vi "Periodic Tasks.vi"(8 "error in":errorcluster) -> ()   [LabVIEW 2015]
doc: "This VI runs in parallel to other tasks. It can contain as many user-defined periodic loops as you need. These can carry out PID or other sorts of timed response."
uses:
  <vilib>/Rock Robotics/WPI/RobotDrive/WPI_RobotDriveMotorSelectorEnum.ctl
  <vilib>/Rock Robotics/WPI/CAN/TalonSRX/WPI_CANTalonSRX_APIFeedbackSelect.ctl
  <vilib>/Rock Robotics/WPI/Utilities/WPI_GetSetVariantRefNum.vi
  Sensors.vi
panel:
  out "x/y":dbl(graph)=0.002857142857142857
  in  "VISA resource name":refnum<visa-resource-name>="FTDI"
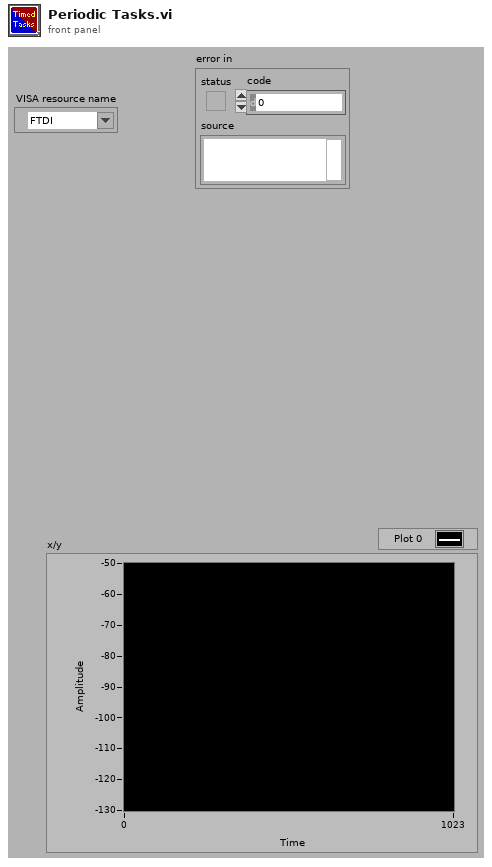
[diagram p1: front panel]
types:
  T1 = typedef "WPI_CANTalonSRX_APIFeedbackSelect.ctl" = enum16{"Digital Quadrature Encoder", "Analog Potentiometer", "Analog Encoder", "Count on Quad-A (Rising-Edge)", "Count on Quad-A (Falling-Edge)", "CTR Magnetic Enc (Absolute)", "CTR Magnetic Enc (Relative)", "Pulse Width"}
  T2 = typedef "WPI_RobotDriveMotorSelectorEnum.ctl" = enum16{"Rear Left Motor", "Rear Right Motor", "Front Left Motor", "Front Right Motor"}
  T3 = typedef "WPI_RobotDriveDevRef.ctl" = cluster{"DevStatus":errorcluster, "Motors[]":T4[], "Square Inputs":bool, "Max Output":dbl}
  T4 = typedef "WPI_MotorControlDeviceRef.ctl" = cluster{"DeviceStatus":errorcluster, "Type":T5, "PWM":cluster{"PWM Channel":T6, "DeadBand":T7}, "CAN":cluster{"Device Number":u8, "Control Mode":T8, "Semaphore":T9, "Max Vout":dbl, "TalonSRX Control Mode":T10}, "Invert":bool}
  T5 = typedef "WPI_MotorControlType.ctl" = enum16{"PWM", "CAN", "CANTalonSRX"}
  T6 = typedef "FPGA_DIOPWMChannel.ctl" = enum8{"PWM 0", "PWM 1", "PWM 2", "PWM 3", "PWM 4", "PWM 5", "PWM 6", "PWM 7", "PWM 8", "PWM 9", "PWM MXP 0", "PWM MXP 1", "PWM MXP 2", "PWM MXP 3", "PWM MXP 4", "PWM MXP 5", "PWM MXP 6", "PWM MXP 7", "PWM MXP 8", "PWM MXP 9", "Invalid"}
  T7 = typedef "WPI_PWMDeadband.ctl" = cluster{"Name":string, "maxPositivePwm":i32, "minPositivePwm":i32, "centerPwm":i32, "maxNegativePwm":i32, "minNegativePwm":i32, "angularRange":u16}
  T8 = typedef "WPI_CANJaguar_ControlMode.ctl" = enum8{"Percent VBus", "Current", "Speed", "Position", "Voltage"}
  T9 = typedef "Semaphore RefNum" = refnum<k1>
  T10 = typedef "WPI_CANTalonSRX_APIControlMode.ctl" = enum8{"Percent VBus", "Speed", "Position", "Slave", "Unchanged / Invalid", "Voltage Compensation", "Current", "Motion Profile"}
  T11 = typedef "WPI_JoystickDevRef.ctl" = cluster{"Device":T12}
  T12 = typedef "WPI_JoystickDeviceEnum.ctl" = enum16{"USB 0", "USB 1", "USB 2", "USB 3", "USB 4", "USB 5"}
  T13 = cluster{"JoystickDevRef":T11, "RobotDriveDevRef":T3}
  T14 = typedef "WPI_AccelerometerDevRef.ctl" = cluster{"DevStatus":errorcluster, "Scaling":T15, "Analog Channels":T16, "I2C Bus":T18, "SPI Bus":T19, "Accel Range":T20, "ADXL Axes":T21, "Handle":i32, "Device Address":u8, "Accel Type":enum16{"Analog", "ADXL345 I2C", "ADXL345 SPI", "Internal", "ADXL362 SPI"}}
  T15 = typedef "WPI_AccelerometerScaling.ctl" = cluster{"Gain (VoltsPerG)":dbl, "Center Voltage":dbl}
  T16 = typedef "WPI_AccelerometerAnalogChannels.ctl" = cluster{"X-Axis":T17, "Y-Axis":T17, "Z-Axis":T17}
  T17 = typedef "FPGA_AIChannel.ctl" = enum8{"AI 0", "AI 1", "AI 2", "AI 3", "AI MXP 0", "AI MXP 1", "AI MXP 2", "AI MXP 3", "Invalid"}
  T18 = typedef "i2c_bus.ctl" = enum16{"I2C On-Board", "I2C MXP", "Invalid"}
  T19 = typedef "spi_bus.ctl" = enum16{"SPI On-Board, CS0", "SPI On-Board, CS1", "SPI On-Board, CS2", "SPI On-Board, CS3", "SPI MXP", "Invalid"}
  T20 = typedef "ADXL345 Range.ctl" = u8
  T21 = typedef "WPI_AccelerometerADXL345 Axes.ctl" = cluster{"X-Axis":bool, "Y-Axis":bool, "Z-Axis":bool}
  T22 = typedef "WPI_CANTalonSRX_GlobalStatus.ctl" = cluster{"Applied Throttle":dbl, "Module Enabled":bool, "CAN Error":errorcluster, "Closed Loop Error":dbl, "Forward Limit Switch Closed":bool, "Reverse Limit Switch Closed":bool, "Sensor Position":dbl, "Sensor Velocity":dbl, "Current":dbl, "Sticky Fault - Over Temp":bool, "Sticky Fault - Under Voltage":bool, "Sticky Fault - Forward Limit":bool, "Sticky Fault - Reverse Limit":bool, "Sticky Fault - Forward Soft Limit":bool, "Sticky Fault - Reverse Soft Limit":bool, "Brake is Enabled":bool, "Encoder Position":dbl, "Encoder Velocity":dbl, "Encoder Index Count":dbl, "Encoder A Pin State":bool, "Encoder B Pin State":bool, "Encoder Index Pin State":bool, "Analog In":dbl, "Analog In Velocity":dbl, "Temperature (C)":dbl, "Battery Voltage":dbl, "Control 5 Is Supported":bool, "Current Profile Slot Select":dbl, "Pos Div 8":bool, "Vel Div 4":bool, "Pulse Width Position":i32, "Pulse Width Velocity":i32, "Pulse Width Rise To Rise (us)":i32, "Pulse Width Rise To Fall (us)":i32, "Mot Prof Active Is Under Run":bool, "Mot Prof Active Has Under Run":bool, "Mot Prof Active Is Last":bool, "Mot Prof Active Velocity Only":bool, "Mot Prof Active Is Valid":bool, "Mot Prof Buffer Is Full":bool, "Mot Prof Active Profile Slot Select":i32, "Mot Prof NextID":i32, "Mot Prof Count":i32, "Mot Prof Active Velocity":dbl, "Mot Prof Active Position":dbl, "Mot Prof Output Enable":i32}
  T23 = cluster{"X-Axis":dbl, "Y-Axis":dbl, "Z-Axis":dbl}
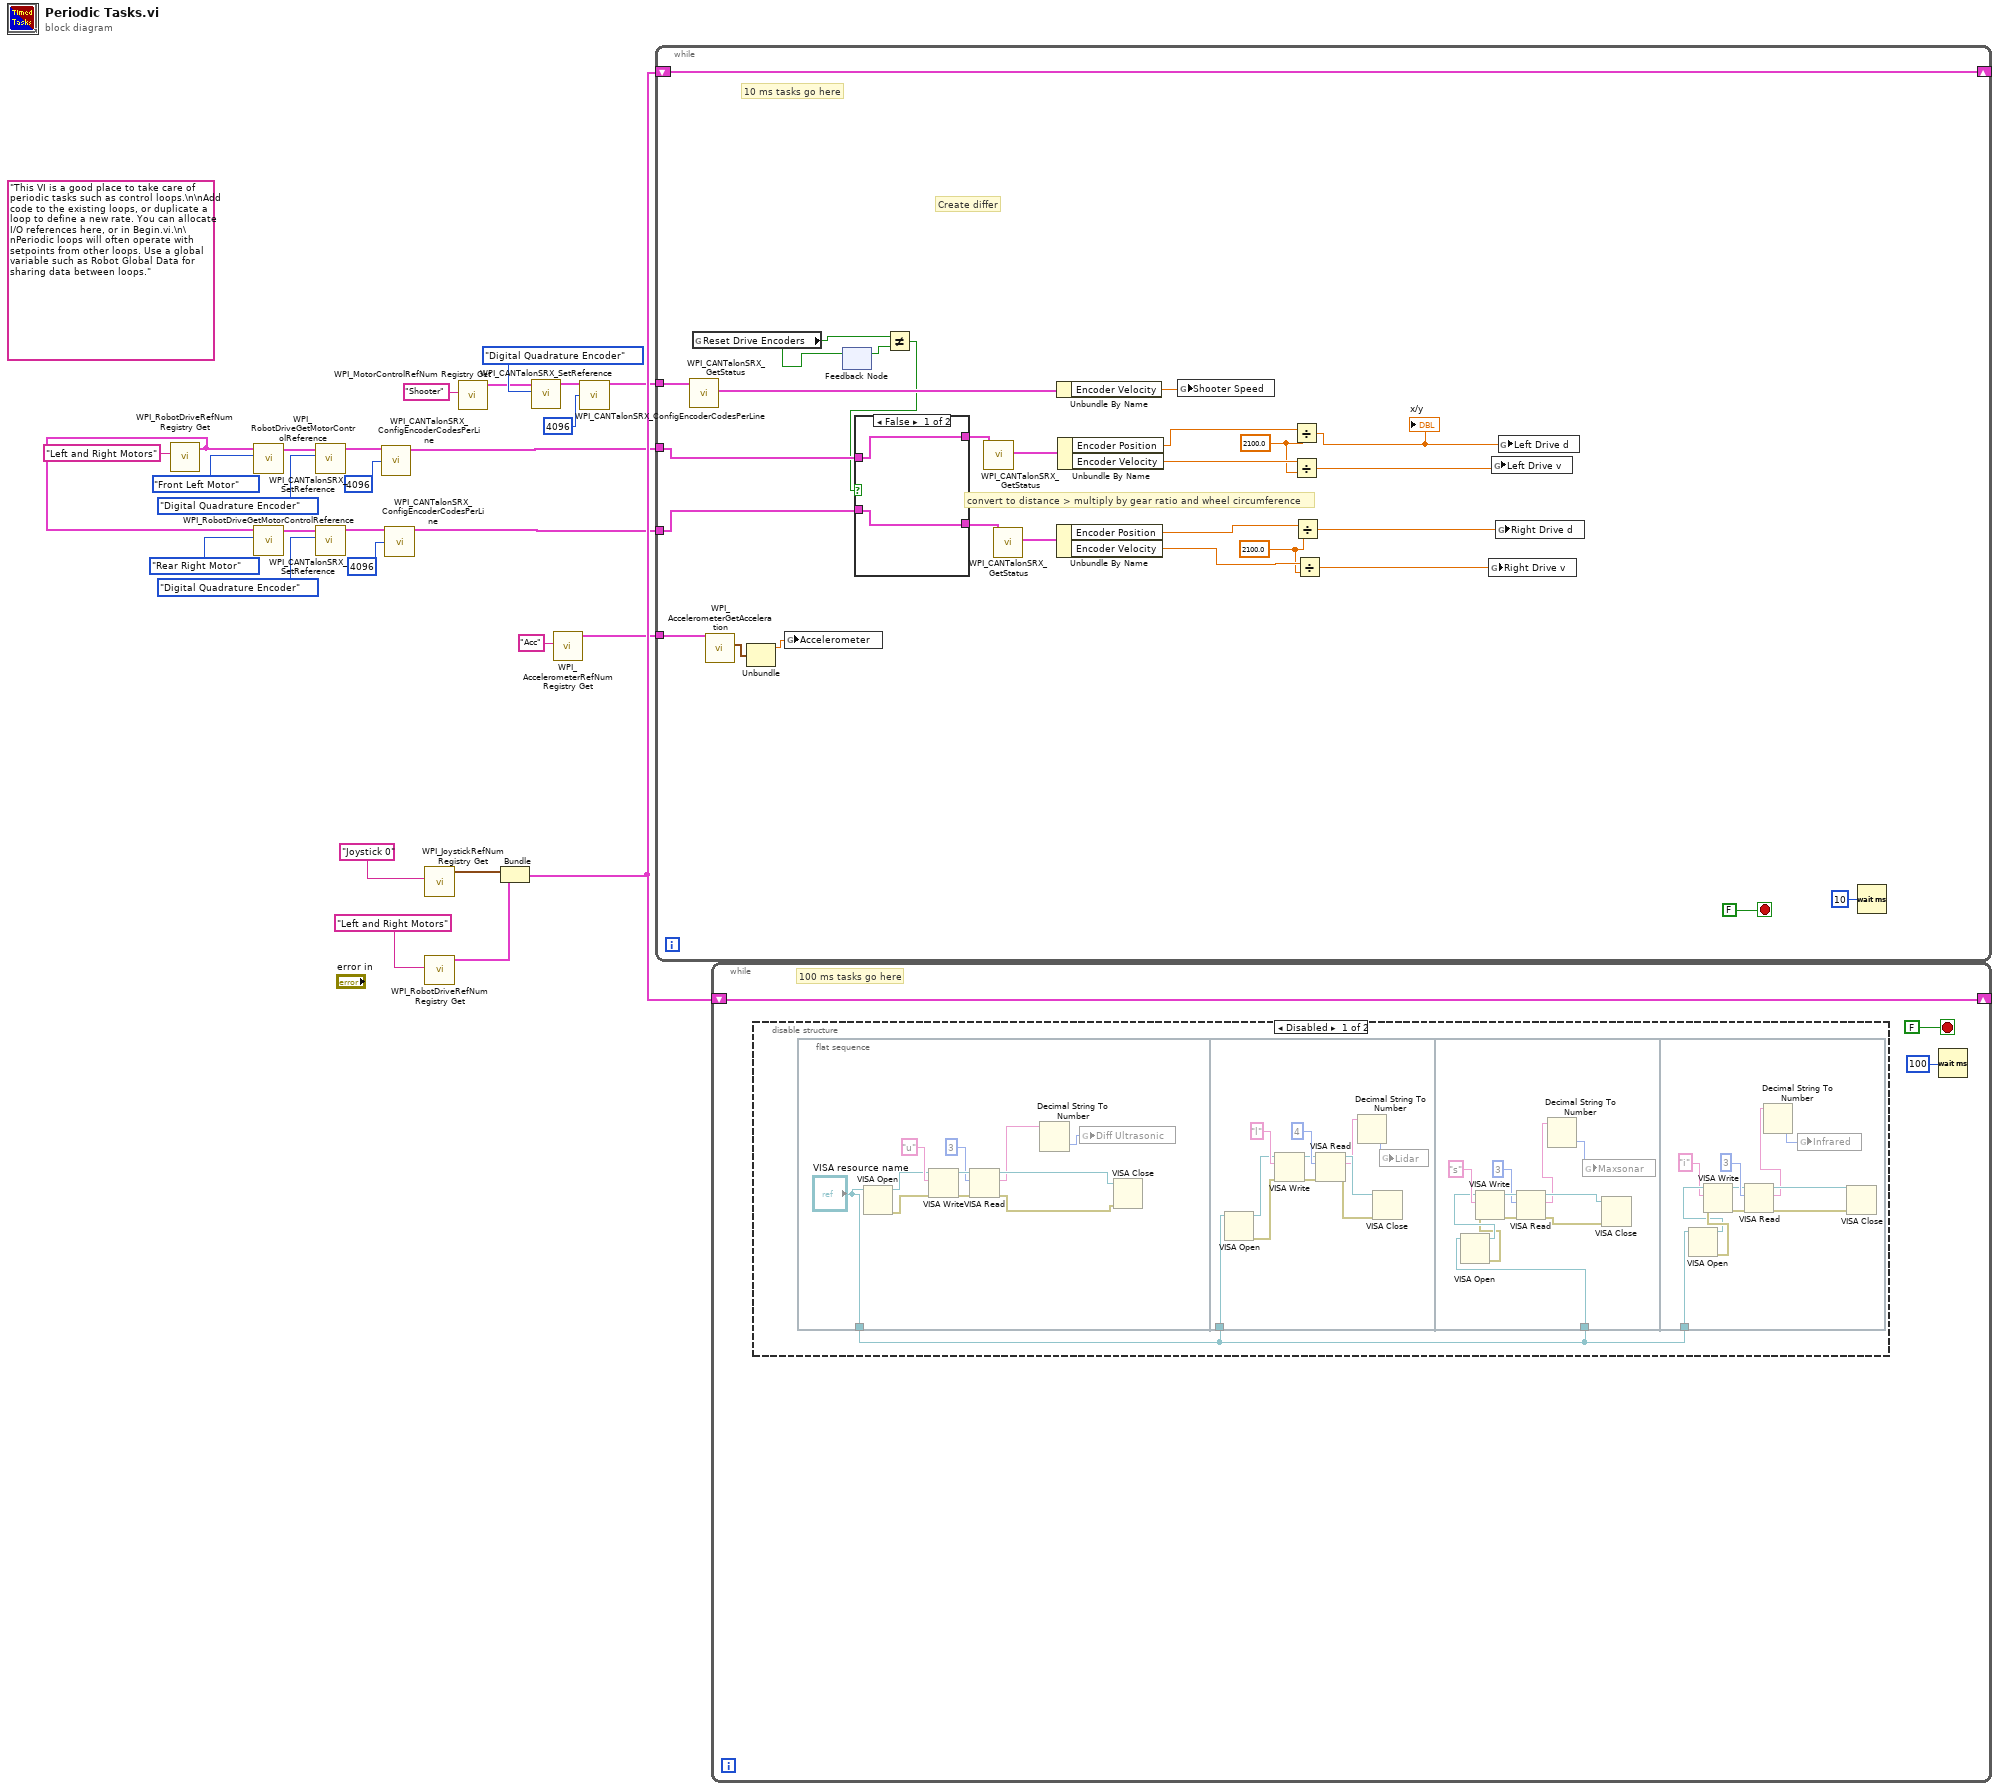
[diagram p0: block diagram]
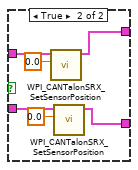
[diagram p3: hidden frame]
diagram:
  (unwired) "This VI is a good place to take care of periodic tasks such as control loops.\n\nAdd code to the existing loops, or duplicate a loop to define a new rate. You can allocate I/O references here, or in Begin.vi.\n\nPeriodic loops will often operate with setpoints from other loops. Use a global variable such as Robot Global Data for sharing data between loops."
  n1 = call <vilib>:"WPI_RobotDriveRefNum Registry Get.vi"("refnum name"="Left and Right Motors") -> ("RobotDriveDevRef"=w8:T3)  [unwired: 9 in, 1 out]
  n2 = call <vilib>:"WPI_RobotDriveGetMotorControlReference.vi"("MotorIndex"=WPI_RobotDriveMotorSelectorEnum."Front Left Motor", "RobotDriveDevRef"=w8) -> ("MotorControlDeviceRef"=w14:T4)  [unwired: 9 out]
  n3 = call <vilib>:"WPI_RobotDriveGetMotorControlReference.vi"("MotorIndex"=WPI_RobotDriveMotorSelectorEnum."Rear Right Motor", "RobotDriveDevRef"=w8) -> ("MotorControlDeviceRef"=w12:T4)  [unwired: 9 out]
  n4 = call <vilib>:"WPI_CANTalonSRX_SetReference.vi"("Feedback Reference"=WPI_CANTalonSRX_APIFeedbackSelect."Digital Quadrature Encoder", "CAN Talon SRX Ref"=w14) -> ("CAN Talon SRX Ref"=w10:T4)  [unwired: 8 in, 1 out]
  n5 = call <vilib>:"WPI_CANTalonSRX_SetReference.vi"("Feedback Reference"=WPI_CANTalonSRX_APIFeedbackSelect."Digital Quadrature Encoder", "CAN Talon SRX Ref"=w12) -> ("CAN Talon SRX Ref"=w6:T4)  [unwired: 8 in, 1 out]
  n6 = call <vilib>:"WPI_CANTalonSRX_ConfigEncoderCodesPerLine.vi"("CAN Talon SRX Ref"=w10, "Number Encoder Lines\n(Counts Per Rotation)"=u32 4096 ("Number Encoder Lines\n(Counts Per Rotation)")) -> ("CAN Talon SRX Ref"=w9:T4)  [unwired: 12 in, 1 out]
  n7 = call <vilib>:"WPI_CANTalonSRX_ConfigEncoderCodesPerLine.vi"("CAN Talon SRX Ref"=w6, "Number Encoder Lines\n(Counts Per Rotation)"=u32 4096 ("Number Encoder Lines\n(Counts Per Rotation)")) -> ("CAN Talon SRX Ref"=w5:T4)  [unwired: 12 in, 1 out]
  n8 = call <vilib>:"WPI_JoystickRefNum Registry Get.vi"("refnum name"="Joystick 0") -> ("JoystickDevRef"=w25:T11)  [unwired: 1 in, 9 out]
  n9 = call <vilib>:"WPI_RobotDriveRefNum Registry Get.vi"("refnum name"="Left and Right Motors") -> ("RobotDriveDevRef"=w24:T3)  [unwired: 1 in, 9 out]
  n10 = call <vilib>:"WPI_MotorControlRefNum Registry Get.vi"("refnum name"="Shooter") -> ("MotorControlDevRef"=w19:T4)  [unwired: 9 in, 1 out]
  n11 = Bundle("JoystickDevRef"=w25, "RobotDriveDevRef"=w24) -> (w23:T13)  [unwired: 1 out]
  n12 = call <vilib>:"WPI_CANTalonSRX_SetReference.vi"("Feedback Reference"=WPI_CANTalonSRX_APIFeedbackSelect."Digital Quadrature Encoder", "CAN Talon SRX Ref"=w19) -> ("CAN Talon SRX Ref"=w18:T4)  [unwired: 8 in, 1 out]
  n13 = call <vilib>:"WPI_AccelerometerRefNum Registry Get.vi"("refnum name"="Acc") -> ("AccelerometerDevRef"=w2:T14)  [unwired: 9 in, 1 out]
  n14 = call <vilib>:"WPI_CANTalonSRX_ConfigEncoderCodesPerLine.vi"("CAN Talon SRX Ref"=w18, "Number Encoder Lines\n(Counts Per Rotation)"=u32 4096 ("Number Encoder Lines\n(Counts Per Rotation)")) -> ("CAN Talon SRX Ref"=w16:T4)  [unwired: 12 in, 1 out]
  n15 = while {
    shift-right: [w54] -> _
    shift-left: w23 -> [w54]
    tunnel: w16 -> [w50]
    tunnel: w9 -> [w49]
    tunnel: w5 -> [w48]
    tunnel: w2 -> [w30]
    stop <- FALSE stop-if-true
    w33 = 2100.0
    w38 = 2100.0 ("y")
    # "Create differ"
    # "convert to distance > multiply by gear ratio and wheel circumference"
    # "10 ms tasks go here"
    n16 = call <vilib>:"WPI_CANTalonSRX_GetStatus.vi"("CAN Talon SRX Ref"=w50) -> ("Talon SRX Status"=w52:T22)  [unwired: 8 in, 2 out]
    n17 = global read "Sensors.vi" "Reset Drive Encoders"() -> (w43:bool)
    n18 = call <vilib>:"WPI_AccelerometerGetAcceleration.vi"("AccelerometerDevRef"=w30) -> ("Accelerations"=w29:T23)  [unwired: 8 in, 2 out]
    n19 = Unbundle(w29) -> ("X-Axis"=w28:dbl)  [unwired: 2 out]
    n20 = global write "Sensors.vi" "Accelerometer"(w28) -> ()
    n21 = feedback-in #1(w43) -> ()
    n22 = feedback #1() -> (w42:bool)  [unwired: 1 in]
    n23 = Not Equal?(x=w43, y=w42) -> (x != y?=w41:bool)
    n24 = case shown="False" w41 {
      tunnel: [w57 w63] -> w45
      tunnel: [w56 w62] -> w47
      tunnel: w49 -> [w57 w61]
      tunnel: w48 -> [w56 w60]
      frame False {
      }
      frame True {
        n25 = call <vilib>:"WPI_CANTalonSRX_SetSensorPosition.vi"("New Sensor Position"=0.0, "CAN Talon SRX Ref"=w61) -> ("CAN Talon SRX Ref"=w63:T4)  [unwired: 8 in, 1 out]
        n26 = call <vilib>:"WPI_CANTalonSRX_SetSensorPosition.vi"("New Sensor Position"=0.0, "CAN Talon SRX Ref"=w60) -> ("CAN Talon SRX Ref"=w62:T4)  [unwired: 8 in, 1 out]
      }
    }
    n27 = call <vilib>:"WPI_CANTalonSRX_GetStatus.vi"("CAN Talon SRX Ref"=w45) -> ("Talon SRX Status"=w44:T22)  [unwired: 8 in, 2 out]
    n28 = call <vilib>:"WPI_CANTalonSRX_GetStatus.vi"("CAN Talon SRX Ref"=w47) -> ("Talon SRX Status"=w46:T22)  [unwired: 8 in, 2 out]
    n29 = Unbundle By Name(w52) -> ("Encoder Velocity"=w51:dbl)
    n30 = Unbundle By Name(w46) -> ("Encoder Position"=w35:dbl, "Encoder Velocity"=w34:dbl)
    n31 = Unbundle By Name(w44) -> ("Encoder Position"=w40:dbl, "Encoder Velocity"=w39:dbl)
    n32 = global write "Sensors.vi" "Shooter Speed"(w51) -> ()
    n33 = Divide(x=w40, y=w38) -> (x/y=w36:dbl)
    "x/y" <- w36
    n34 = Divide(x=w39, y=w38) -> (x/y=w37:dbl)
    n35 = Divide(x=w35, y=w33) -> (x/y=w32:dbl)
    n36 = Divide(x=w34, y=w33) -> (x/y=w31:dbl)
    n37 = global write "Sensors.vi" "Right Drive v"(w31) -> ()
    n38 = global write "Sensors.vi" "Left Drive v"(w37) -> ()
    n39 = global write "Sensors.vi" "Right Drive d"(w32) -> ()
    n40 = global write "Sensors.vi" "Left Drive d"(w36) -> ()
    n41 = Wait (ms)(milliseconds to wait=u32 10) -> ()  [unwired: 1 out]
  }
  n42 = while {
    shift-right: [w64] -> _
    shift-left: w23 -> [w64]
    stop <- FALSE stop-if-true
    # "100 ms tasks go here"
    n43 = disable-structure shown="Disabled" {
      frame Disabled {
        n44 = flat-sequence {
          tunnel: ["VISA resource name"] -> w67
          tunnel: w67 -> [w83]
          tunnel: w67 -> [w96]
          tunnel: w67 -> [w105]
          frame #0 {
            n45 = VISA Open(VISA resource name="VISA resource name") -> (VISA resource name=w71:refnum<visa-resource-name>, error out=w70:errorcluster)  [unwired: 4 in]
            n46 = VISA Write(VISA resource name=w71, write buffer="u", error in (no error)=w70) -> (VISA resource name out=w78:refnum<visa-resource-name>, error out=w77:errorcluster)  [unwired: 1 out]
            n47 = VISA Read(VISA resource name=w78, byte count=u32 3, error in (no error)=w77) -> (VISA resource name out=w74:refnum<visa-resource-name>, read buffer=w72:string, error out=w73:errorcluster)  [unwired: 1 out]
            n48 = Decimal String To Number(string=w72) -> (number=w68:i32)  [unwired: 2 in, 1 out]
            n49 = global write "Sensors.vi" "Diff Ultrasonic"(w68) -> ()
            n50 = VISA Close(VISA resource name=w74, error in (no error)=w73) -> ()  [unwired: 1 out]
          }
          frame #1 {
            n51 = VISA Open(VISA resource name=w83) -> (VISA resource name=w85:refnum<visa-resource-name>, error out=w84:errorcluster)  [unwired: 4 in]
            n52 = VISA Write(VISA resource name=w85, write buffer="l", error in (no error)=w84) -> (VISA resource name out=w86:refnum<visa-resource-name>, error out=w87:errorcluster)  [unwired: 1 out]
            n53 = VISA Read(VISA resource name=w86, byte count=u32 4, error in (no error)=w87) -> (VISA resource name out=w82:refnum<visa-resource-name>, read buffer=w80:string, error out=w81:errorcluster)  [unwired: 1 out]
            n54 = Decimal String To Number(string=w80) -> (number=w79:i32)  [unwired: 2 in, 1 out]
            n55 = VISA Close(VISA resource name=w82, error in (no error)=w81) -> ()  [unwired: 1 out]
            n56 = global write "Sensors.vi" "Lidar"(w79) -> ()
          }
          frame #2 {
            n57 = VISA Open(VISA resource name=w96) -> (VISA resource name=w95:refnum<visa-resource-name>, error out=w94:errorcluster)  [unwired: 4 in]
            n58 = VISA Write(VISA resource name=w95, write buffer="s", error in (no error)=w94) -> (VISA resource name out=w100:refnum<visa-resource-name>, error out=w99:errorcluster)  [unwired: 1 out]
            n59 = VISA Read(VISA resource name=w100, byte count=u32 3, error in (no error)=w99) -> (VISA resource name out=w93:refnum<visa-resource-name>, read buffer=w91:string, error out=w92:errorcluster)  [unwired: 1 out]
            n60 = Decimal String To Number(string=w91) -> (number=w90:i32)  [unwired: 2 in, 1 out]
            n61 = global write "Sensors.vi" "Maxsonar"(w90) -> ()
            n62 = VISA Close(VISA resource name=w93, error in (no error)=w92) -> ()  [unwired: 1 out]
          }
          frame #3 {
            n63 = VISA Open(VISA resource name=w105) -> (VISA resource name=w110:refnum<visa-resource-name>, error out=w111:errorcluster)  [unwired: 4 in]
            n64 = VISA Write(VISA resource name=w110, write buffer="i", error in (no error)=w111) -> (VISA resource name out=w106:refnum<visa-resource-name>, error out=w107:errorcluster)  [unwired: 1 out]
            n65 = VISA Read(VISA resource name=w106, byte count=u32 3, error in (no error)=w107) -> (VISA resource name out=w104:refnum<visa-resource-name>, read buffer=w102:string, error out=w103:errorcluster)  [unwired: 1 out]
            n66 = Decimal String To Number(string=w102) -> (number=w101:i32)  [unwired: 2 in, 1 out]
            n67 = global write "Sensors.vi" "Infrared"(w101) -> ()
            n68 = VISA Close(VISA resource name=w104, error in (no error)=w103) -> ()  [unwired: 1 out]
          }
        }
      }
      frame Enabled {
      }
    }
    n69 = Wait (ms)(milliseconds to wait=u32 100) -> ()  [unwired: 1 out]
  }
